vi "SPARK Get Closed Loop Config Gains.vi"(6 "Closed Loop Slot (0)":T1 items=["Slot 0", "Slot 1", "Slot 2", "Slot 3"], 8 "error in":errorcluster, 11 "MotorControlDeviceRef in":T4={"DeviceStatus"={"status"=FALSE, "code"=0, "source"=""}, "Type"=enum."PWM", "PWM"={"PWM Channel"=enum."Invalid", "DeadBand"={"Name"="", "maxPositivePwm"=0, "minPositivePwm"=0, "centerPwm"=0, "maxNegativePwm"=0, "minNegativePwm"=0, "angularRange"=0}}, "CAN"={"Device Number"=0, "SetOutput VI Ref"=variant(refnum<vi> refnum), "GetOutput VI Ref"=variant(refnum<vi> refnum), "Enable VI Ref"=variant(refnum<vi> refnum), "Disable VI Ref"=variant(refnum<vi> refnum), "Data"=variant}, "Invert"=FALSE, "DIO PWM"={"PWM \"Enable\" Channel"=enum."Invalid", "DIOChannel"=enum."Invalid", "PWM Rate"=0.0}}) -> (0 "error out":errorcluster, 1 "Feed Forward Gains":T2={"kV"=nan, "kS"=nan, "kA"=nan, "kG"=nan, "kCos"=nan, "kCosRatio"=nan}, 2 "PID Gains":T3={"kP"=nan, "kI"=nan, "kD"=nan}, 3 "MotorControlDeviceRef out":T4={"DeviceStatus"={"status"=FALSE, "code"=0, "source"=""}, "Type"=enum."PWM", "PWM"={"PWM Channel"=enum."Invalid", "DeadBand"={"Name"="", "maxPositivePwm"=0, "minPositivePwm"=0, "centerPwm"=0, "maxNegativePwm"=0, "minNegativePwm"=0, "angularRange"=0}}, "CAN"={"Device Number"=0, "SetOutput VI Ref"=variant(refnum<vi> refnum), "GetOutput VI Ref"=variant(refnum<vi> refnum), "Enable VI Ref"=variant(refnum<vi> refnum), "Disable VI Ref"=variant(refnum<vi> refnum), "Data"=variant}, "Invert"=FALSE, "DIO PWM"={"PWM \"Enable\" Channel"=enum."Invalid", "DIOChannel"=enum."Invalid", "PWM Rate"=0.0}}, 5 "Allowed Closed Loop Error":dbl)   [LabVIEW 2023]
doc: "Get the configure PID and feed forward gains of the closed loop controller of the SPARK."
uses:
  <vilib>/Rock Robotics/WPI/MotorControl/WPI_MotorControlDeviceRef.ctl
  <vilib>/Rock Robotics/WPI/MotorControl/WPI_MotorControlType.ctl
  <vilib>/Rock Robotics/SystemInterfaces/DIO/FPGA_DIOPWMChannel.ctl
  <vilib>/Rock Robotics/WPI/PWM/WPI_PWMDeadband.ctl
  <vilib>/Rock Robotics/SystemInterfaces/DIO/FPGA_DIOChannel.ctl
  Typedef/SPARK PID Gains.ctl
  Typedef/SPARK Feed Forward Gains.ctl
  Typedef/SPARK Closed Loop Slot.ctl
  Typedef/SPARK Parameter ID.ctl
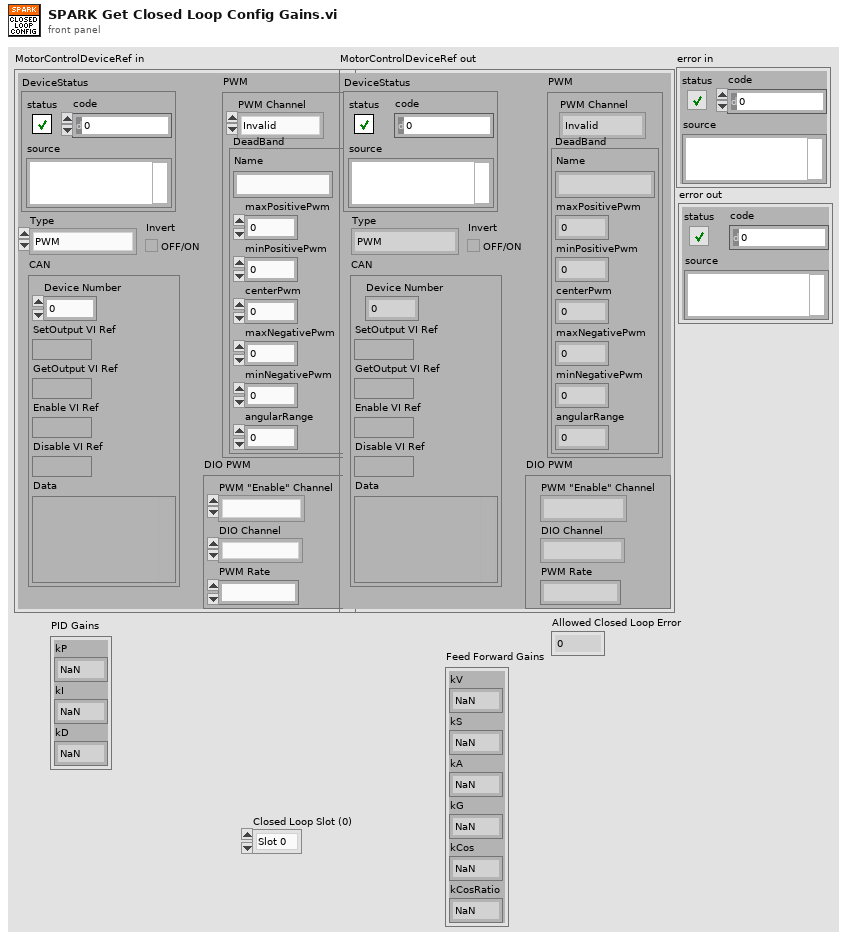
[diagram p1: front panel]
types:
  T1 = typedef "SPARK Closed Loop Slot.ctl" = u16
  T2 = typedef "SPARK Feed Forward Gains.ctl" = cluster{"kV":dbl, "kS":dbl, "kA":dbl, "kG":dbl, "kCos":dbl, "kCosRatio":dbl}
  T3 = typedef "SPARK PID Gains.ctl" = cluster{"kP":dbl, "kI":dbl, "kD":dbl}
  T4 = typedef "WPI_MotorControlDeviceRef.ctl" = cluster{"DeviceStatus":errorcluster, "Type":T5, "PWM":cluster{"PWM Channel":T6, "DeadBand":T7}, "CAN":cluster{"Device Number":u8, "SetOutput VI Ref":variant, "GetOutput VI Ref":variant, "Enable VI Ref":variant, "Disable VI Ref":variant, "Data":variant}, "Invert":bool, "DIO PWM":cluster{"PWM \"Enable\" Channel":T6, "DIOChannel":T8, "PWM Rate":dbl}}
  T5 = typedef "WPI_MotorControlType.ctl" = enum16{"PWM", "CAN", "DIO PWM"}
  T6 = typedef "FPGA_DIOPWMChannel.ctl" = enum8{"PWM 0", "PWM 1", "PWM 2", "PWM 3", "PWM 4", "PWM 5", "PWM 6", "PWM 7", "PWM 8", "PWM 9", "PWM MXP 0", "PWM MXP 1", "PWM MXP 2", "PWM MXP 3", "PWM MXP 4", "PWM MXP 5", "PWM MXP 6", "PWM MXP 7", "PWM MXP 8", "PWM MXP 9", "Invalid"}
  T7 = typedef "WPI_PWMDeadband.ctl" = cluster{"Name":string, "maxPositivePwm":i32, "minPositivePwm":i32, "centerPwm":i32, "maxNegativePwm":i32, "minNegativePwm":i32, "angularRange":u16}
  T8 = typedef "FPGA_DIOChannel.ctl" = enum8{"DIO 0", "DIO 1", "DIO 2", "DIO 3", "DIO 4", "DIO 5", "DIO 6", "DIO 7", "DIO 8", "DIO 9", "DIO MXP 0", "DIO MXP 1", "DIO MXP 2", "DIO MXP 3", "DIO MXP 4", "DIO MXP 5", "DIO MXP 6", "DIO MXP 7", "DIO MXP 8", "DIO MXP 9", "DIO MXP 10", "DIO MXP 11", "DIO MXP 12", "DIO MXP 13", "DIO MXP 14", "DIO MXP 15", "SPI Port CS1", "SPI Port CS2", "SPI Port CS3", "SPI Port MISO", "SPI Port MOSI", "Invalid"}
  T9 = typedef "SPARK Parameter ID.ctl" = enum16{"kCanID", "kInputMode", "kMotorType", "kCommAdvance", "kSensorType", "kCtrlType", "kIdleMode", "kInputDeadband", "kLegacyFeedbackSensorPID0", "kClosedLoopControlSensor", "kPolePairs", "kCurrentChop", "kCurrentChopCycles", "kP_0", "kI_0", "kD_0", "kV_0", "kIZone_0", "kDFilter_0", "kOutputMin_0", "kOutputMax_0", "kP_1", "kI_1", "kD_1", "kV_1", "kIZone_1", "kDFilter_1", "kOutputMin_1", "kOutputMax_1", "kP_2", "kI_2", "kD_2", "kV_2", "kIZone_2", "kDFilter_2", "kOutputMin_2", "kOutputMax_2", "kP_3", "kI_3", "kD_3", "kV_3", "kIZone_3", "kDFilter_3", "kOutputMin_3", "kOutputMax_3", "kInverted", "kOutputRatio", "kSerialNumberLow", "kSerialNumberMid", "kSerialNumberHigh", "kLimitSwitchFwdPolarity", "kLimitSwitchRevPolarity", "kHardLimitFwdEn", "kHardLimitRevEn", "kSoftLimitFwdEn", "kSoftLimitRevEn", "kRampRate", "kFollowerID", "kFollowerConfig", "kSmartCurrentStallLimit", "kSmartCurrentFreeLimit", "kSmartCurrentConfig", "kSmartCurrentReserved", "kMotorKv", "kMotorR", "kMotorL", "kMotorRsvd1", "kMotorRsvd2", "kMotorRsvd3", "kEncoderCountsPerRev", "kEncoderAverageDepth", "kEncoderSampleDelta", "kEncoderInverted", "kEncoderRsvd1", "kClosedLoopVoltageMode", "kCompensatedNominalVoltage", "kSmartMotionMaxVelocity_0", "kSmartMotionMaxAccel_0", "kSmartMotionMinVelOutput_0", "kSmartMotionAllowedClosedLoopError_0", "kSmartMotionAccelStrategy_0", "kSmartMotionMaxVelocity_1", "kSmartMotionMaxAccel_1", "kSmartMotionMinVelOutput_1", "kSmartMotionAllowedClosedLoopError_1", "kSmartMotionAccelStrategy_1", "kSmartMotionMaxVelocity_2", "kSmartMotionMaxAccel_2", "kSmartMotionMinVelOutput_2", "kSmartMotionAllowedClosedLoopError_2", "kSmartMotionAccelStrategy_2", "kSmartMotionMaxVelocity_3", "kSmartMotionMaxAccel_3", "kSmartMotionMinVelOutput_3", "kSmartMotionAllowedClosedLoopError_3", "kSmartMotionAccelStrategy_3", "kIMaxAccum_0", "kAllowedClosedLoopError_0", "kSlot3Placeholder2_0", "kSlot3Placeholder3_0", "kIMaxAccum_1", "kAllowedClosedLoopError_1", "kSlot3Placeholder2_1", "kSlot3Placeholder3_1", "kIMaxAccum_2", "kAllowedClosedLoopError_2", "kSlot3Placeholder2_2", "kSlot3Placeholder3_2", "kIMaxAccum_3", "kAllowedClosedLoopError_3", "kSlot3Placeholder2_3", "kSlot3Placeholder3_3", "kPositionConversionFactor", "kVelocityConversionFactor", "kClosedLoopRampRate", "kSoftLimitFwd", "kSoftLimitRev", "kSoftLimitRsvd0", "kSoftLimitRsvd1", "kAnalogPositionConversion", "kAnalogVelocityConversion", "kAnalogAverageDepth", "kAnalogSensorMode", "kAnalogInverted", "kAnalogSampleDelta", "kAnalogRsvd0", "kAnalogRsvd1", "kDataPortConfig", "kAltEncoderCountsPerRev", "kAltEncoderAverageDepth", "kAltEncoderSampleDelta", "kAltEncoderInverted", "kAltEncoderPositionConversion", "kAltEncoderVelocityConversion", "kAltEncoderRsvd0", "kAltEncoderRsvd1", "kHallSensorSampleRate", "kHallSensorAverageDepth", "kNumParameters", "kDutyCyclePositionFactor", "kDutyCycleVelocityFactor", "kDutyCycleInverted", "kDutyCycleSensorMode", "kDutyCycleAverageDepth", "kDutyCycleSampleDelta", "kDutyCycleOffsetv1p6p2", "kDutyCycleRsvd0", "kDutyCycleRsvd1", "kDutyCycleRsvd2", "kPositionPIDWrapEnable", "kPositionPIDMinInput", "kPositionPIDMaxInput", "kDutyCycleZeroCentered", "kDutyCyclePrescalar", "kDutyCycleOffset", "kProductId", "kDeviceMajorVersion", "kDeviceMinorVersion", "kStatus0Period", "kStatus1Period", "kStatus2Period", "kStatus3Period", "kStatus4Period", "kStatus5Period", "kStatus6Period", "kStatus7Period", "kMAXMotionCruiseVelocity_0", "kMAXMotionMaxAccel_0", "kMAXMotionMaxJerk_0", "kMAXMotionAllowedProfileError_0", "kMAXMotionPositionMode_0", "kMAXMotionCruiseVelocity_1", "kMAXMotionMaxAccel_1", "kMAXMotionMaxJerk_1", "kMAXMotionAllowedProfileError_1", "kMAXMotionPositionMode_1", "kMAXMotionCruiseVelocity_2", "kMAXMotionMaxAccel_2", "kMAXMotionMaxJerk_2", "kMAXMotionAllowedProfileError_2", "kMAXMotionPositionMode_2", "kMAXMotionCruiseVelocity_3", "kMAXMotionMaxAccel_3", "kMAXMotionMaxJerk_3", "kMAXMotionAllowedProfileError_3", "kMAXMotionPositionMode_3", "kForceEnableStatus0", "kForceEnableStatus1", "kForceEnableStatus2", "kForceEnableStatus3", "kForceEnableStatus4", "kForceEnableStatus5", "kForceEnableStatus6", "kForceEnableStatus7", "kFollowerModeLeaderId", "kFollowerModeIsInverted", "kDutyCycleEncoderStartPulseUs", "kDutyCycleEncoderEndPulseUs", "kParamTableVersion", "kStatus8Period", "kForceEnableStatus8", "kLimitSwitchPositionSensor", "kLimitSwitchForwardPosition", "kLimitSwitchReversePosition", "kS_0", "kA_0", "kG_0", "kCos_0", "kCosRatio_0", "kS_1", "kA_1", "kG_1", "kCos_1", "kCosRatio_1", "kS_2", "kA_2", "kG_2", "kCos_2", "kCosRatio_2", "kS_3", "kA_3", "kG_3", "kCos_3", "kCosRatio_3", "kStatus9Period", "kForceEnableStatus9"}
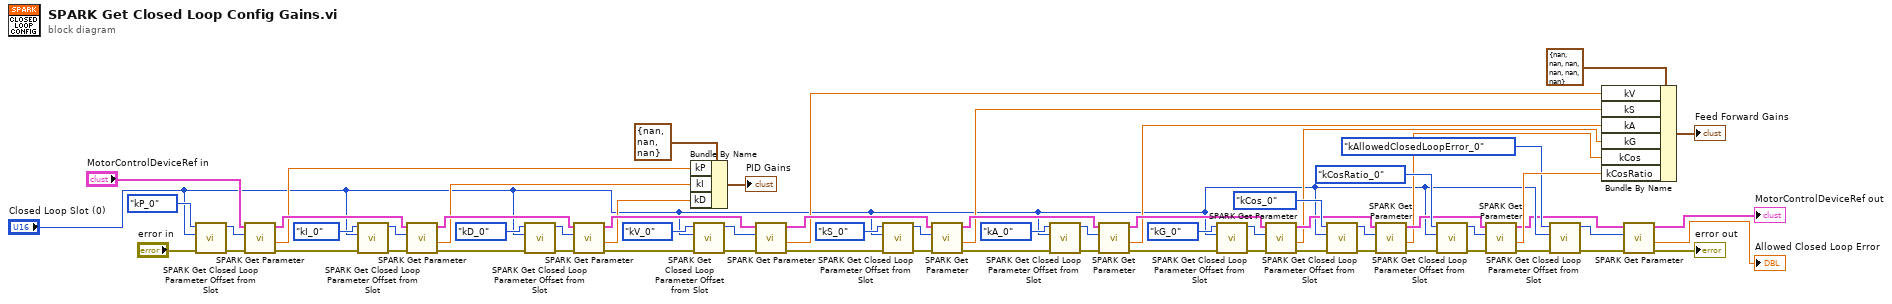
[diagram p0: block diagram]
diagram:
  n1 = call "SPARK Get Closed Loop Parameter Offset from Slot.vi"("error in (no error)"="error in", "Closed Loop Slot"="Closed Loop Slot (0)", "Parameter ID in"=SPARK_Parameter_ID."kP_0") -> ("error out"=w59:errorcluster, "Parameter ID out"=w64:T9)  [unwired: 7 in]
  n2 = call "SPARK Get Parameter.vi"("error in (no error)"=w59, "Parameter ID in"=w64, "MotorControlDeviceRef in"="MotorControlDeviceRef in") -> ("error out"=w58:errorcluster, "float"=w45:dbl, "MotorControlDeviceRef"=w53:T4)  [unwired: 3 in, 3 out]
  n3 = call "SPARK Get Closed Loop Parameter Offset from Slot.vi"("error in (no error)"=w58, "Closed Loop Slot"="Closed Loop Slot (0)", "Parameter ID in"=SPARK_Parameter_ID."kI_0") -> ("error out"=w57:errorcluster, "Parameter ID out"=w63:T9)  [unwired: 7 in]
  n4 = call "SPARK Get Parameter.vi"("error in (no error)"=w57, "Parameter ID in"=w63, "MotorControlDeviceRef in"=w53) -> ("error out"=w56:errorcluster, "float"=w46:dbl, "MotorControlDeviceRef"=w54:T4)  [unwired: 3 in, 3 out]
  n5 = call "SPARK Get Closed Loop Parameter Offset from Slot.vi"("error in (no error)"=w56, "Closed Loop Slot"="Closed Loop Slot (0)", "Parameter ID in"=SPARK_Parameter_ID."kD_0") -> ("error out"=w55:errorcluster, "Parameter ID out"=w62:T9)  [unwired: 7 in]
  n6 = call "SPARK Get Parameter.vi"("error in (no error)"=w55, "Parameter ID in"=w62, "MotorControlDeviceRef in"=w54) -> ("error out"=w49:errorcluster, "float"=w47:dbl, "MotorControlDeviceRef"=w52:T4)  [unwired: 3 in, 3 out]
  n7 = Bundle By Name(cluster=T3 {"kP"=nan, "kI"=nan, "kD"=nan} ("PID Gains"), "kP"=w45, "kI"=w46, "kD"=w47) -> (→"PID Gains":T3)
  n8 = call "SPARK Get Closed Loop Parameter Offset from Slot.vi"("error in (no error)"=w49, "Closed Loop Slot"="Closed Loop Slot (0)", "Parameter ID in"=SPARK_Parameter_ID."kV_0") -> ("error out"=w48:errorcluster, "Parameter ID out"=w51:T9)  [unwired: 7 in]
  n9 = call "SPARK Get Parameter.vi"("error in (no error)"=w48, "Parameter ID in"=w51, "MotorControlDeviceRef in"=w52) -> ("error out"=w17:errorcluster, "float"=w10:dbl, "MotorControlDeviceRef"=w26:T4)  [unwired: 3 in, 3 out]
  n10 = call "SPARK Get Closed Loop Parameter Offset from Slot.vi"("error in (no error)"=w17, "Closed Loop Slot"="Closed Loop Slot (0)", "Parameter ID in"=SPARK_Parameter_ID."kS_0") -> ("error out"=w41:errorcluster, "Parameter ID out"=w39:T9)  [unwired: 7 in]
  n11 = call "SPARK Get Parameter.vi"("error in (no error)"=w41, "Parameter ID in"=w39, "MotorControlDeviceRef in"=w26) -> ("error out"=w18:errorcluster, "float"=w11:dbl, "MotorControlDeviceRef"=w25:T4)  [unwired: 3 in, 3 out]
  n12 = call "SPARK Get Closed Loop Parameter Offset from Slot.vi"("error in (no error)"=w18, "Closed Loop Slot"="Closed Loop Slot (0)", "Parameter ID in"=SPARK_Parameter_ID."kA_0") -> ("error out"=w36:errorcluster, "Parameter ID out"=w38:T9)  [unwired: 7 in]
  n13 = call "SPARK Get Parameter.vi"("error in (no error)"=w36, "Parameter ID in"=w38, "MotorControlDeviceRef in"=w25) -> ("error out"=w19:errorcluster, "float"=w12:dbl, "MotorControlDeviceRef"=w24:T4)  [unwired: 3 in, 3 out]
  n14 = call "SPARK Get Closed Loop Parameter Offset from Slot.vi"("error in (no error)"=w19, "Closed Loop Slot"="Closed Loop Slot (0)", "Parameter ID in"=SPARK_Parameter_ID."kG_0") -> ("error out"=w35:errorcluster, "Parameter ID out"=w33:T9)  [unwired: 7 in]
  n15 = call "SPARK Get Parameter.vi"("error in (no error)"=w35, "Parameter ID in"=w33, "MotorControlDeviceRef in"=w24) -> ("error out"=w20:errorcluster, "float"=w13:dbl, "MotorControlDeviceRef"=w23:T4)  [unwired: 3 in, 3 out]
  n16 = call "SPARK Get Closed Loop Parameter Offset from Slot.vi"("error in (no error)"=w20, "Closed Loop Slot"="Closed Loop Slot (0)", "Parameter ID in"=SPARK_Parameter_ID."kCos_0") -> ("error out"=w30:errorcluster, "Parameter ID out"=w32:T9)  [unwired: 7 in]
  n17 = call "SPARK Get Parameter.vi"("error in (no error)"=w30, "Parameter ID in"=w32, "MotorControlDeviceRef in"=w23) -> ("error out"=w21:errorcluster, "float"=w14:dbl, "MotorControlDeviceRef"=w22:T4)  [unwired: 3 in, 3 out]
  n18 = call "SPARK Get Closed Loop Parameter Offset from Slot.vi"("error in (no error)"=w21, "Closed Loop Slot"="Closed Loop Slot (0)", "Parameter ID in"=SPARK_Parameter_ID."kCosRatio_0") -> ("error out"=w29:errorcluster, "Parameter ID out"=w27:T9)  [unwired: 7 in]
  n19 = call "SPARK Get Parameter.vi"("error in (no error)"=w29, "Parameter ID in"=w27, "MotorControlDeviceRef in"=w22) -> ("error out"=w5:errorcluster, "float"=w15:dbl, "MotorControlDeviceRef"=w4:T4)  [unwired: 3 in, 3 out]
  n20 = call "SPARK Get Closed Loop Parameter Offset from Slot.vi"("error in (no error)"=w5, "Closed Loop Slot"="Closed Loop Slot (0)", "Parameter ID in"=SPARK_Parameter_ID."kAllowedClosedLoopError_0") -> ("error out"=w8:errorcluster, "Parameter ID out"=w9:T9)  [unwired: 7 in]
  n21 = Bundle By Name(cluster=T2 {"kV"=nan, "kS"=nan, "kA"=nan, "kG"=nan, "kCos"=nan, "kCosRatio"=nan} ("Feed Forward Gains"), "kV"=w10, "kS"=w11, "kA"=w12, "kG"=w13, "kCos"=w14, "kCosRatio"=w15) -> (→"Feed Forward Gains":T2)
  n22 = call "SPARK Get Parameter.vi"("error in (no error)"=w8, "Parameter ID in"=w9, "MotorControlDeviceRef in"=w4) -> ("error out"=→"error out":errorcluster, "float"=→"Allowed Closed Loop Error":dbl, "MotorControlDeviceRef"=→"MotorControlDeviceRef out":T4)  [unwired: 3 in, 3 out]
